vi "Verify HTML Tables and Digraph.vi"() -> (3 "test passed":bool)   [LabVIEW 2015]
uses:
  GraphViz Mapping Visualizer.lvlib
  <vilib>/NI/Tag Bus/tag/Data Type.ctl
  <vilib>/NI/Tag Bus/tag/tag descriptor.lvclass
panel:
  out "digraph output":string
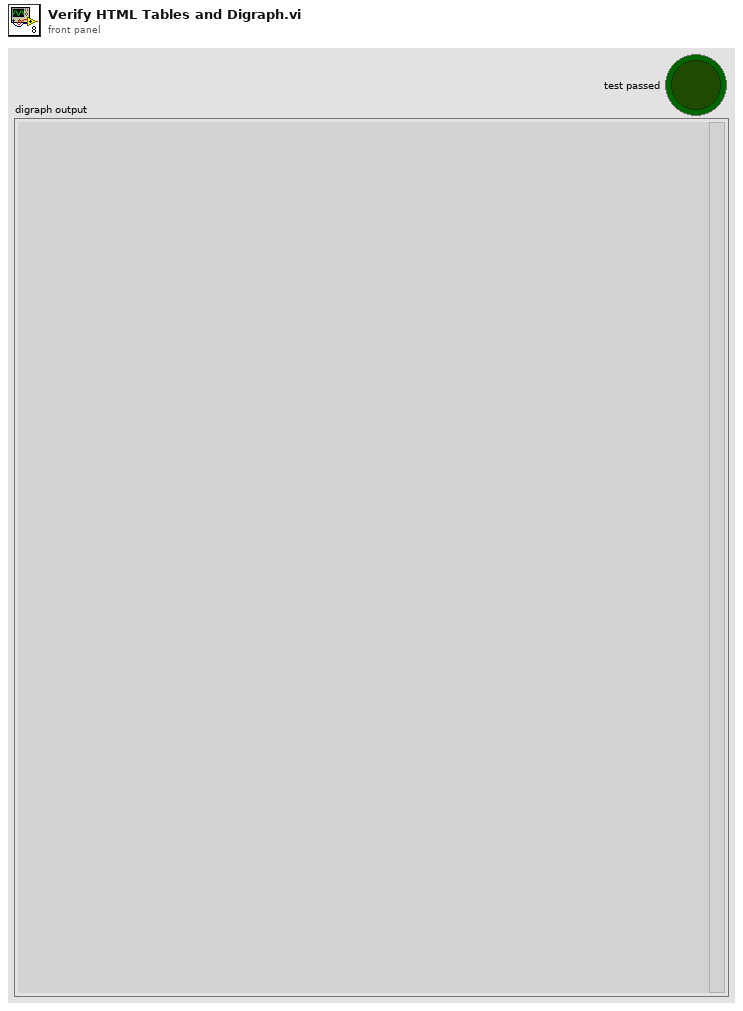
[diagram p1: front panel]
types:
  T1 = typedef "tag bus.lvlib/tag descriptor.lvclass/Data Type.ctl" = enum16{"Double", "Single", "I64", "I32", "I16", "I8", "U64", "U32", "U16", "U8", "Boolean", "String", "Array of Double", "Array of Single", "Array of I64", "Array of I32", "Array of I16", "Array of I8", "Array of U64", "Array of U32", "Array of U16", "Array of U8", "Array of Boolean", "Array of String"}
  T2 = cluster{"name":string, "data type":T1, "writer":string, "readers":string[]}[]
  T3 = cluster{"Instance ID":string, "name":string, "default value string":string, "index":i32}[]
  T4 = typedef "GraphViz Mapping Visualizer.lvlib/Channel to Port Pair.ctl" = cluster{"Channel Name":string, "Node:Port":string}
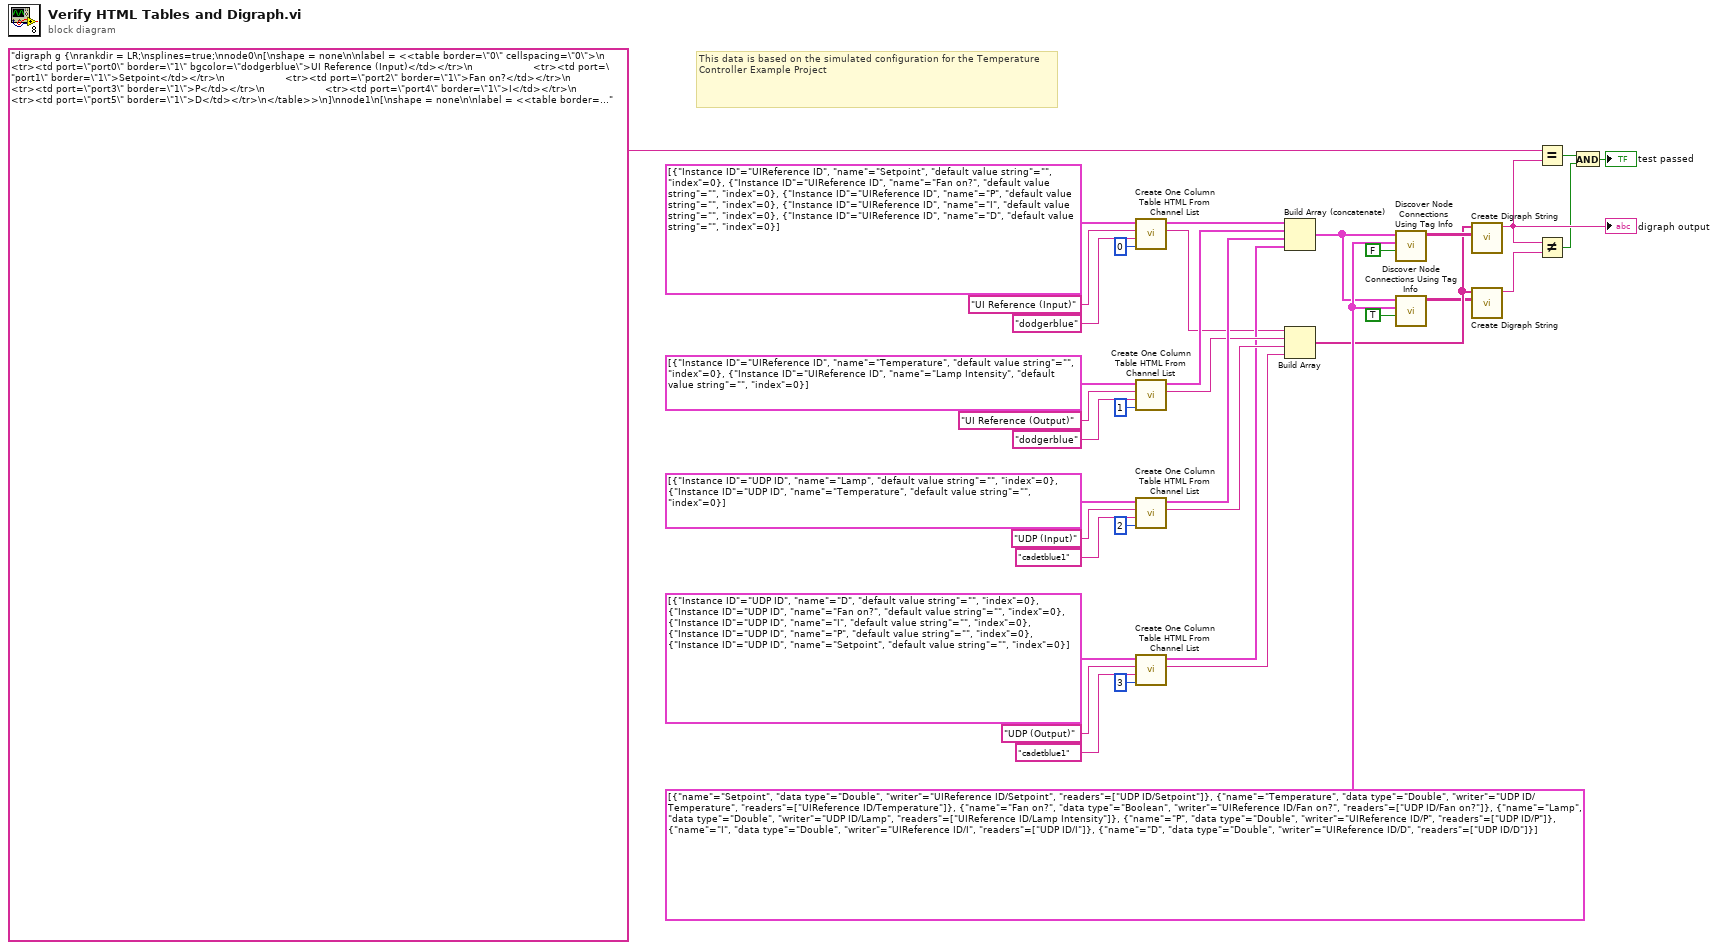
[diagram p0: block diagram]
diagram:
  w4 = T2 [{"name"="Setpoint", "data type"=enum."Double", "writer"="UIReference ID/Setpoint", "readers"=["UDP ID/Setpoint"]}, {"name"="Temperature", "data type"=enum."Double", "writer"="UDP ID/Temperature", "readers"=["UIReference ID/Temperature"]}, {"name"="Fan on?", "data type"=enum."Boolean", "writer"="UIReference ID/Fan on?", "readers"=["UDP ID/Fan on?"]}, {"name"="Lamp", "data type"=enum."Double", "writer"="UDP ID/Lamp", "readers"=["UIReference ID/Lamp Intensity"]}, {"name"="P", "data type"=enum."Double", "writer"="UIReference ID/P", "readers"=["UDP ID/P"]}, {"name"="I", "data type"=enum."Double", "writer"="UIReference ID/I", "readers"=["UDP ID/I"]}, {"name"="D", "data type"=enum."Double", "writer"="UIReference ID/D", "readers"=["UDP ID/D"]}] ("tag info")
  # "This data is based on the simulated configuration for the Temperature Controller Example Project"
  n1 = call "Create One Column Table HTML From Channel List.vi"("Node#"=0, "Color"="dodgerblue" ("Title"), "Title"="UI Reference (Input)", "display strings and indices"=T3 [{"Instance ID"="UIReference ID", "name"="Setpoint", "default value string"="", "index"=0}, {"Instance ID"="UIReference ID", "name"="Fan on?", "default value string"="", "index"=0}, {"Instance ID"="UIReference ID", "name"="P", "default value string"="", "index"=0}, {"Instance ID"="UIReference ID", "name"="I", "default value string"="", "index"=0}, {"Instance ID"="UIReference ID", "name"="D", "default value string"="", "index"=0}]) -> ("Table HTML"=w15:string, "Channel and Node Pairs"=w36:T4[])  [unwired: 6 in]
  n2 = call "Create One Column Table HTML From Channel List.vi"("Node#"=1, "Color"="dodgerblue" ("Title"), "Title"="UI Reference (Output)", "display strings and indices"=T3 [{"Instance ID"="UIReference ID", "name"="Temperature", "default value string"="", "index"=0}, {"Instance ID"="UIReference ID", "name"="Lamp Intensity", "default value string"="", "index"=0}]) -> ("Table HTML"=w32:string, "Channel and Node Pairs"=w33:T4[])  [unwired: 6 in]
  n3 = call "Create One Column Table HTML From Channel List.vi"("Node#"=2, "Color"="cadetblue1" ("Title"), "Title"="UDP (Input)", "display strings and indices"=T3 [{"Instance ID"="UDP ID", "name"="Lamp", "default value string"="", "index"=0}, {"Instance ID"="UDP ID", "name"="Temperature", "default value string"="", "index"=0}]) -> ("Table HTML"=w37:string, "Channel and Node Pairs"=w35:T4[])  [unwired: 6 in]
  n4 = call "Create One Column Table HTML From Channel List.vi"("Node#"=3, "Color"="cadetblue1" ("Title"), "Title"="UDP (Output)", "display strings and indices"=T3 [{"Instance ID"="UDP ID", "name"="D", "default value string"="", "index"=0}, {"Instance ID"="UDP ID", "name"="Fan on?", "default value string"="", "index"=0}, {"Instance ID"="UDP ID", "name"="I", "default value string"="", "index"=0}, {"Instance ID"="UDP ID", "name"="P", "default value string"="", "index"=0}, {"Instance ID"="UDP ID", "name"="Setpoint", "default value string"="", "index"=0}]) -> ("Table HTML"=w30:string, "Channel and Node Pairs"=w31:T4[])  [unwired: 6 in]
  n5 = Build Array (concatenate)(w36, w33, w35, w31) -> (w3:T4[])
  n6 = Build Array(w15, w32, w37, w30) -> (w2:string[])
  n7 = call "Discover Node Connections Using Tag Info.vi"("Show Tag Labels?"=FALSE, "tag info"=w4, "channel and node pairs"=w3) -> ("node connections"=w6:string[][])  [unwired: 8 in]
  n8 = call "Discover Node Connections Using Tag Info.vi"("Show Tag Labels?"=TRUE, "tag info"=w4, "channel and node pairs"=w3) -> ("node connections"=w1:string[][])  [unwired: 8 in]
  n9 = call "Create Digraph String.vi"("node connections"=w6, "tables html"=w2) -> ("digraph output"=w12:string)  [unwired: 9 in]
  "digraph output" <- w12
  n10 = call "Create Digraph String.vi"("node connections"=w1, "tables html"=w2) -> ("digraph output"=w11:string)  [unwired: 9 in]
  n11 = Equal?(x="digraph g {\nrankdir = LR;\nsplines=true;\nnode0\n[\nshape = none\n\nlabel = <<table border=\"0\" cellspacing=\"0\">\n                    <tr><td port=\"port0\" border=\"1\" bgcolor=\"dodgerblue\">UI Reference (Input)</td></tr>\n                    <tr><td port=\"port1\" border=\"1\">Setpoint</td></tr>\n                    <tr><td port=\"port2\" border=\"1\">Fan on?</td></tr>\n                    <tr><td port=\"port3\" border=\"1\">P</td></tr>\n                    <tr><td port=\"port4\" border=\"1\">I</td></tr>\n                    <tr><td port=\"port5\" border=\"1\">D</td></tr>\n</table>>\n]\nnode1\n[\nshape = none\n\nlabel = <<table border=\"0\" cellspacing=\"0\">\n                    <tr><td port=\"port0\" border=\"1\" bgcolor=\"dodgerblue\">UI Reference (Output)</td></tr>\n                    <tr><td port=\"port1\" border=\"1\">Temperature</td></tr>\n                    <tr><td port=\"port2\" border=\"1\">Lamp Intensity</td></tr>\n</table>>\n]\nnode2\n[\nshape = none\n\nlabel = <<table border=\"0\" cellspacing=\"0\">\n                    <tr><td port=\"port0\" border=\"1\" bgcolor=\"cadetblue1\">UDP (Input)</td></tr>\n                    <tr><td port=\"port1\" border=\"1\">Lamp</td></tr>\n                    <tr><td port=\"port2\" border=\"1\">Temperature</td></tr>\n</table>>\n]\nnode3\n[\nshape = none\n\nlabel = <<table border=\"0\" cellspacing=\"0\">\n                    <tr><td port=\"port0\" border=\"1\" bgcolor=\"cadetblue1\">UDP (Output)</td></tr>\n                    <tr><td port=\"port1\" border=\"1\">D</td></tr>\n                    <tr><td port=\"port2\" border=\"1\">Fan on?</td></tr>\n                    <tr><td port=\"port3\" border=\"1\">I</td></tr>\n                    <tr><td port=\"port4\" border=\"1\">P</td></tr>\n                    <tr><td port=\"port5\" border=\"1\">Setpoint</td></tr>\n</table>>\n]\nnode0:port1 -> node3:port5 [color=\"orange\"]\r\nnode2:port2 -> node1:port1 [color=\"orange\"]\r\nnode0:port2 -> node3:port2 [color=\"green\"]\r\nnode2:port1 -> node1:port2 [color=\"orange\"]\r\nnode0:port3 -> node3:port4 [color=\"orange\"]\r\nnode0:port4 -> node3:port3 [color=\"orange\"]\r\nnode0:port5 -> node3:port1 [color=\"orange\"]\r\n}" ("String"), y=w12) -> (x = y?=w9:bool)
  n12 = Not Equal?(x=w12, y=w11) -> (x != y?=w10:bool)
  n13 = And(x=w9, y=w10) -> (x .and. y?=→"test passed":bool)
